vi "Asynch Simple U3 U6.vi"() -> ()   [LabVIEW 2021]
panel:
  out "Device Type Found":string
  out "Actual Baud Rate":dbl
  out "BaudFactor":i32
  in  "Desired Baud Rate":i32=9600
  out "Bytes in Read Buffer before read":i32
  in  "# Bytes To Write":i32=4 min=1 max=50
  out "U8 Array Read":u8[](array[numeric])=[99, 99, 99, 99, 99, 99, 99, 99, 99, 99, 99, 99, 99, 99, 99, 99, 99, 99, 99, 99, 99, 99, 99, 99, 99, 99, 99, 99, 99, 99, 99, 99]
  in  "U8 Array Write":u8[](array[numeric])=[170, 240, 170, 240]
  out "Error Message":string
  out "error out":errorcluster
  # "You can short TX to RX for loopback testing.  TX/RX appear after any timers and counters\non the U3 and U6, but this VI disables all timers and counters.\n\nTX       U3-FIO4, U6-FIO0\nRX       U3-FIO5, U6-FIO1\n\nThis simple VI does a write, waits 1 second, then returns whatever was read in that time.\nIf you short TX to RX, then you will read back the same bytes that you write."
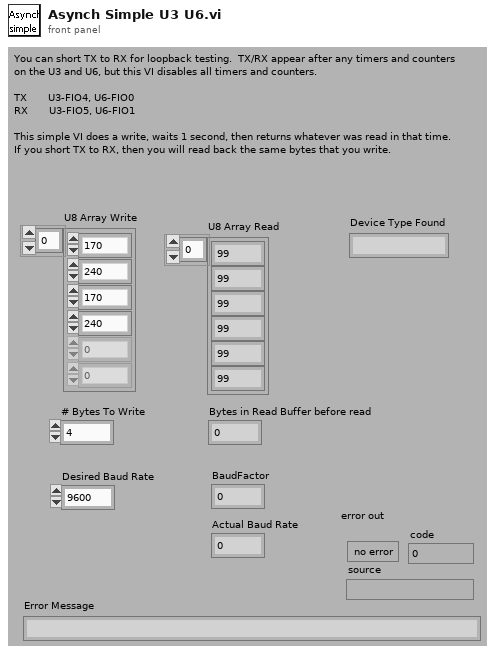
[diagram p1: front panel]
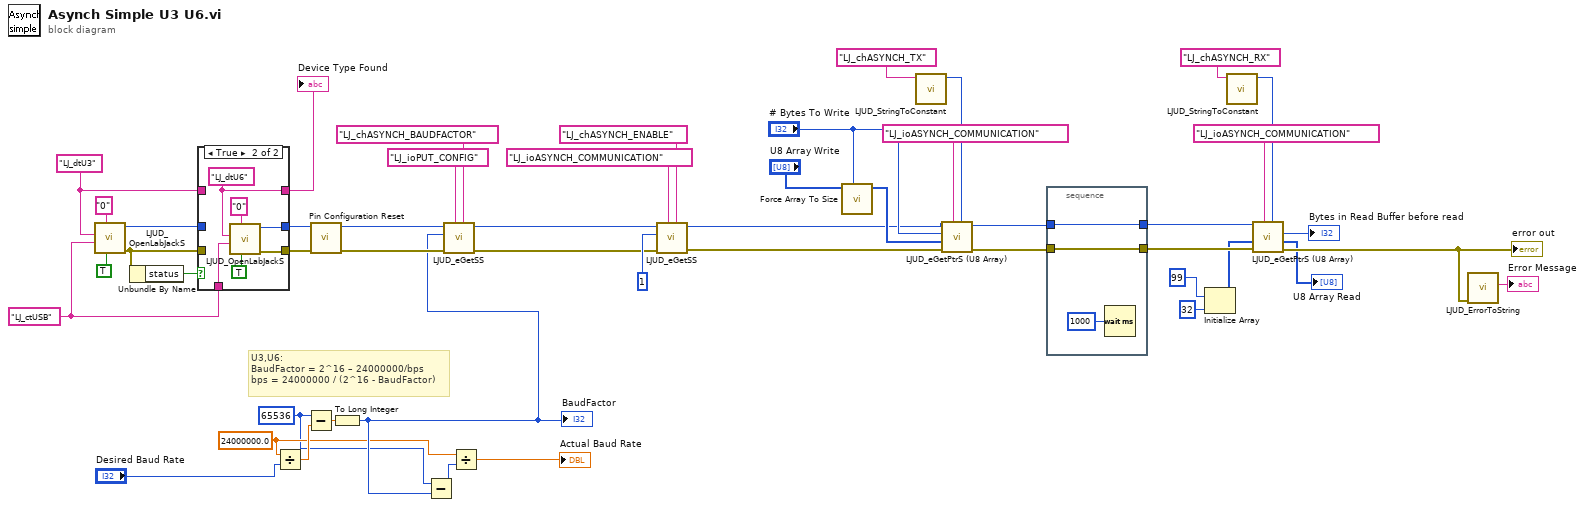
[diagram p0: block diagram]
diagram:
  w1 = 65536 ("x")
  w2 = 24000000.0 ("x")
  w36 = "LJ_ctUSB" ("ConnectionType")
  w6 = "LJ_dtU3" ("DeviceType")
  # "U3,U6:\nBaudFactor = 2^16 – 24000000/bps \nbps = 24000000 / (2^16 - BaudFactor)"
  n1 = call "LJUD_OpenLabJackS.vi"("FirstFound"=TRUE, "Address"="0", "ConnectionType"=w36, "DeviceType"=w6) -> ("error out"=w40:errorcluster, "Handle"=w38:i32)  [unwired: 5 in, 1 out]
  n2 = Unbundle By Name(w40) -> ("status"=w11:bool)
  n3 = case shown="True" w11 {
    tunnel: w40 -> [w52 _]
    tunnel: [w52 w55] -> w39
    tunnel: w38 -> [w51 _]
    tunnel: [w51 w54] -> w37
    tunnel: w36 -> [_ w56]
    tunnel: [w50 w53] -> w7
    tunnel: w6 -> [w50 _]
    frame False {
    }
    frame True {
      w53 = "LJ_dtU6" ("DeviceType")
      n4 = call "LJUD_OpenLabJackS.vi"("FirstFound"=TRUE, "Address"="0", "ConnectionType"=w56, "DeviceType"=w53) -> ("error out"=w55:errorcluster, "Handle"=w54:i32)  [unwired: 5 in, 1 out]
    }
  }
  "Device Type Found" <- w7
  n5 = Divide(x=w2, y="Desired Baud Rate") -> (x/y=w5:dbl)
  n6 = Subtract(x=w1, y=w5) -> (x-y=w4:dbl)
  n7 = call "Pin Configuration Reset.vi"("error in"=w39, "Handle In"=w37) -> ("error out"=w42:errorcluster, "Handle Out"=w41:i32)  [unwired: 8 in]
  n8 = To Long Integer(number=w4) -> (32bit integer=w8:i32)
  "BaudFactor" <- w8
  n9 = Subtract(x=w1, y=w8) -> (x-y=w3:i32)
  n10 = call "LJUD_eGetSS.vi"("Channel"="LJ_chASYNCH_BAUDFACTOR", "IOType"="LJ_ioPUT_CONFIG", "error in"=w42, "Value Write"=w8, "Handle In"=w41) -> ("error out"=w30:errorcluster, "Handle Out"=w29:i32)  [unwired: 4 in, 1 out]
  n11 = Divide(x=w2, y=w3) -> (x/y=→"Actual Baud Rate":dbl)
  n12 = call "LJUD_eGetSS.vi"("Channel"="LJ_chASYNCH_ENABLE", "IOType"="LJ_ioASYNCH_COMMUNICATION", "error in"=w30, "Value Write"=1 ("Value"), "Handle In"=w29) -> ("error out"=w19:errorcluster, "Handle Out"=w18:i32)  [unwired: 4 in, 1 out]
  n13 = call "Force Array To Size.vi"("# Elements"="# Bytes To Write", "I32 Array In"="U8 Array Write") -> ("I32 Array Out"=w43:i32[])  [unwired: 6 in, 3 out]
  n14 = call "LJUD_StringToConstant.vi"("String"="LJ_chASYNCH_TX" ("Channel")) -> ("Constant Number"=w25:i32)  [unwired: 9 in, 1 out]
  n15 = call "LJUD_eGetPtrS (U8 Array).vi"("Channel"=w25, "IOType"="LJ_ioASYNCH_COMMUNICATION", "error in"=w19, "U8 Array Write"=w43, "Value"="# Bytes To Write", "Handle In"=w18) -> ("error out"=w20:errorcluster, "Handle Out"=w17:i32)  [unwired: 2 in, 2 out]
  n16 = stacked-sequence {
    tunnel: [w61] -> w15
    tunnel: w20 -> [w61]
    tunnel: [w60] -> w16
    tunnel: w17 -> [w60]
    frame #0 {
      n17 = Wait (ms)(milliseconds to wait=u32 1000) -> ()  [unwired: 1 out]
    }
  }
  n18 = Initialize Array(u8 99 ("Element Data"), 32 ("Dimension Size")) -> (w14:u8[])
  n19 = call "LJUD_StringToConstant.vi"("String"="LJ_chASYNCH_RX" ("Channel")) -> ("Constant Number"=w24:i32)  [unwired: 9 in, 1 out]
  n20 = call "LJUD_eGetPtrS (U8 Array).vi"("Channel"=w24, "IOType"="LJ_ioASYNCH_COMMUNICATION", "error in"=w15, "U8 Array Write"=w14, "Handle In"=w16) -> ("error out"=w22:errorcluster, "U8 Array Read"=→"U8 Array Read":u8[], "Value"=→"Bytes in Read Buffer before read":i32)  [unwired: 3 in, 1 out]
  "error out" <- w22
  n21 = call "LJUD_ErrorToString.vi"("error in"=w22) -> ("String"=→"Error Message":string)  [unwired: 10 in]
